vi "DeviceIsOpen.vi"(6 "Delay between send and receive [ms]":i32=100, 8 "error in (no error)":errorcluster, 11 "SCD in":refnum<class "SCD.lvclass">) -> (0 "error out":errorcluster, 1 "ID":i32, 2 "device is open?":bool, 3 "SCD out":refnum<class "SCD.lvclass">)   [LabVIEW 2023, in "SCD.lvclass"]
doc: "Returns true if selected SpectrAcq3 is open."
uses:
  SCD.lvclass
  GenericDevice/GenericDevice.lvclass
panel:
  # "Connector Pane"
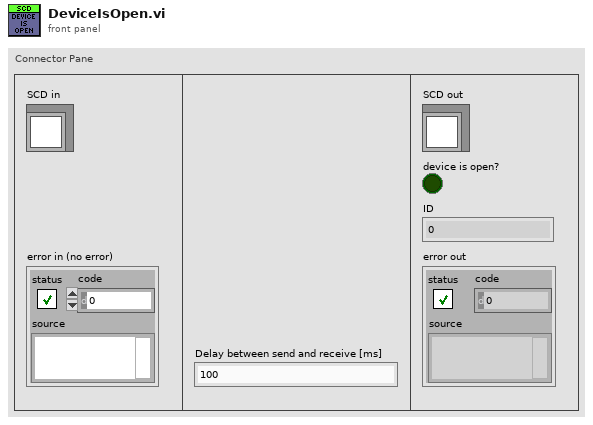
[diagram p1: front panel]
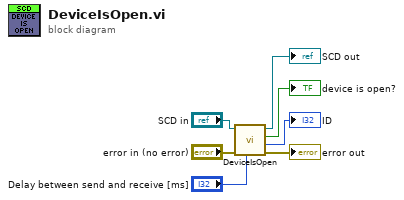
[diagram p0: block diagram]
diagram:
  n1 = call-parent "DeviceIsOpen.vi"("Delay between send and receive [ms]"="Delay between send and receive [ms]", "error in (no error)"="error in (no error)", "GenericDevice in"="SCD in") -> ("error out"=→"error out":errorcluster, "ID"=→"ID":i32, "device is open?"=→"device is open?":bool, "GenericDevice out"=→"SCD out":refnum<class "SCD.lvclass">)  [unwired: 5 in]
